vi "Return_EnFlo_Tunnel_to_Neutral.vi"(3 "Mode":T5, 5 "Traverse line In":T2 {"Carrier_2 Q (l/min)" format="%#.2f"; "Row Duration (mins)" format="%#.1f"; "Row No" min=0; "Trace Gas Concentration (%)" min=0.0 format="%#_4f"; "Carrier_1 Q (l/min)" format="%#.2f"; "Tunnel Speed" format="%#.2f"; "Start X" format="%#.2f"; "Start Y" format="%#.2f"; "Start Z" format="%#.2f"; "End X" format="%#.2f"; "End Y" format="%#.2f"; "End Z" format="%#.2f"; "Averaging time (min)" min=0.0 format="%#.2f"}) -> (0 "Error Message":string, 1 "Status":T1, 2 "Traverse line Out":T2 {"Carrier_2 Q (l/min)" format="%#.2f"; "Row Duration (mins)" format="%#.1f"; "Row No" min=0; "Trace Gas Concentration (%)" min=0.0 format="%#_4f"; "Carrier_1 Q (l/min)" format="%#.2f"; "Tunnel Speed" format="%#.2f"; "Start X" format="%#.2f"; "Start Y" format="%#.2f"; "Start Z" format="%#.2f"; "End X" format="%#.2f"; "End Y" format="%#.2f"; "End Z" format="%#.2f"; "Averaging time (min)" min=0.0 format="%#.2f"})   [LabVIEW 2016]
uses:
  Gen Trav/Traverse_cluster.ctl
  Gen Trav/Spacing.ctl
  Controls/Multi_run_mode.ctl
  Controls/User_Specific_mode.ctl
  Gen Trav/Multi_Run_Status.ctl
  ADAM Client/Sub VIs/ADAM Controls/Update_scan_value.ctl
  ADAM Client/Sub VIs/ADAM Controls/Channel_names.ctl
  ADAM Client/Sub VIs/ADAM Controls/Client_Source_Status.ctl
  Globals/Trav_pos_global.vi
panel:
  out "Chilled water supply temp":dbl(graph)
  # "X           Y            Z"
  # "Start"
  # "End"
  # "X           Y            Z"
  # "Start"
  # "End"
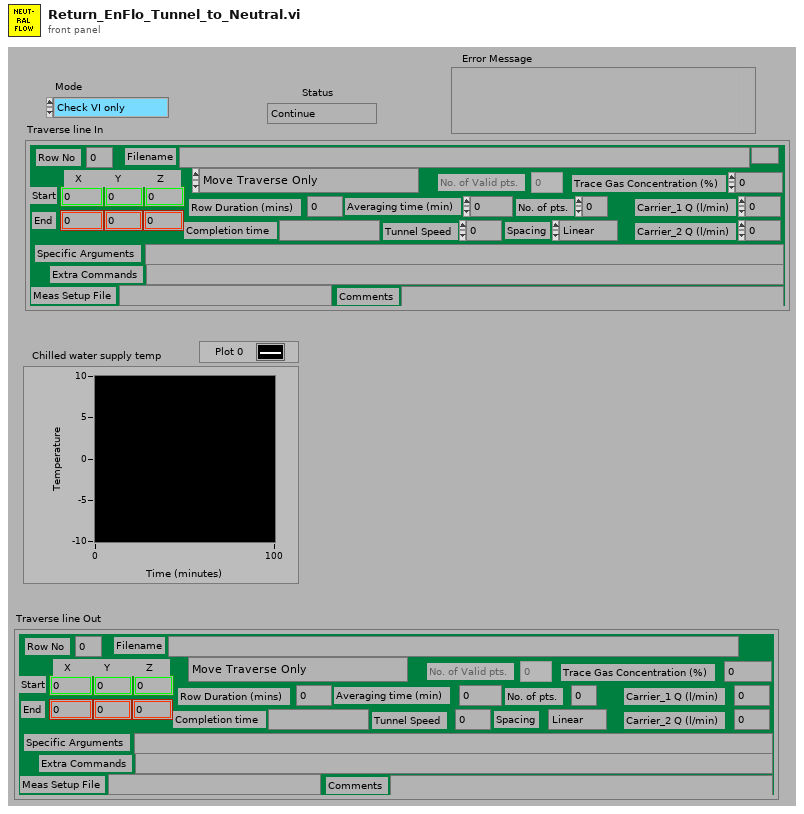
[diagram p1: front panel]
types:
  T1 = typedef "Multi_Run_Status.ctl" = enum16{"Continue", "Jump to Next Point", "Jump to Next Row", "Jump To Fall Back", "Terminate Run"}
  T2 = typedef "Traverse_cluster.ctl" = cluster{"Start X":sgl, "Start Y":sgl, "Start Z":sgl, "End X":sgl, "End Y":sgl, "End Z":sgl, "No. of pts.":i32, "Spacing":T3, "Filename":path, "Tunnel Speed":dbl, "Averaging time (min)":dbl, "Extra Commands":string, "Carrier_1 Q (l/min)":dbl, "Carrier_2 Q (l/min)":dbl, "Trace Gas Concentration (%)":dbl, "Specific Arguments":string, "Comments":string, "Row No":i32, "Row Type Selector":T4, "Completion time":string, "Row Duration (mins)":dbl, "No. of Valid pts.":i32, "Meas Setup File":string}
  T3 = typedef "Spacing.ctl" = enum16{"Linear", "Log", "Gauss", "Specified", "N/A"}
  T4 = typedef "Multi_run_mode.ctl" = enum16{"Move Traverse Only", "Set Tunnel Speed Only", "Set Source Only", "Set Measurement Conditions", "Single Measurement", "Vertical Profile", "Lateral Profile", "Longitudinal Profile", "Explore Volume", "Multi-Axis Profile", "Auto Calibrate", "Meas Fast FID Bkgnd", "Check Beam Power", "Scanning Valve Measurement", "Run VI Named:", "Set ADAM Ch", "Wait (minutes)", "Send Message", "Synchronize With:", "Fall Back to this Row", "Turn Off Row Repeating", "Blank Row", "Traverse 3D Volume"}
  T5 = typedef "User_Specific_mode.ctl" = enum16{"Check VI only", "Run VI"}
  T6 = typedef "Update_scan_value.ctl" = cluster{"Channel Name":string, "New Value":dbl}
  T7 = typedef "Channel_names.ctl" = enum16{"Active Only", "Active + Off", "All Channels"}
  T8 = typedef "Client_Source_Status.ctl" = enum16{"Not Using", "Using", "Must Have"}
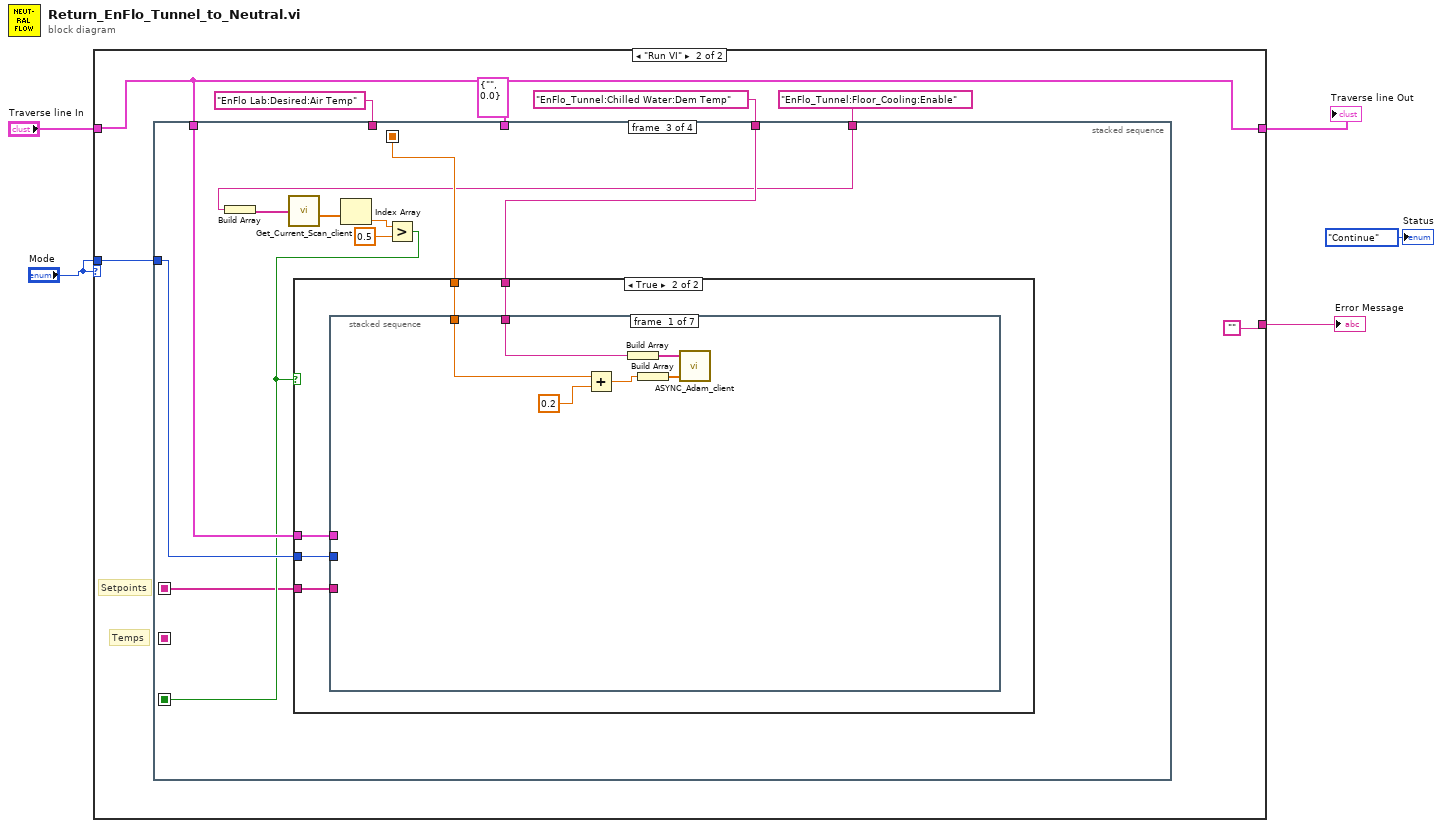
[diagram p0: block diagram]
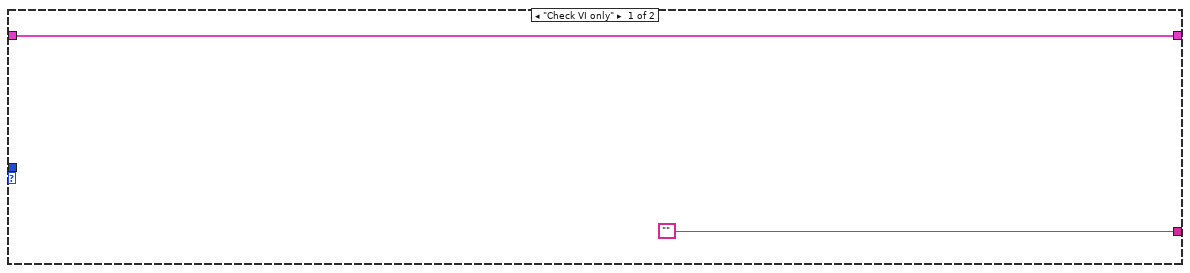
[diagram p2: hidden frame]
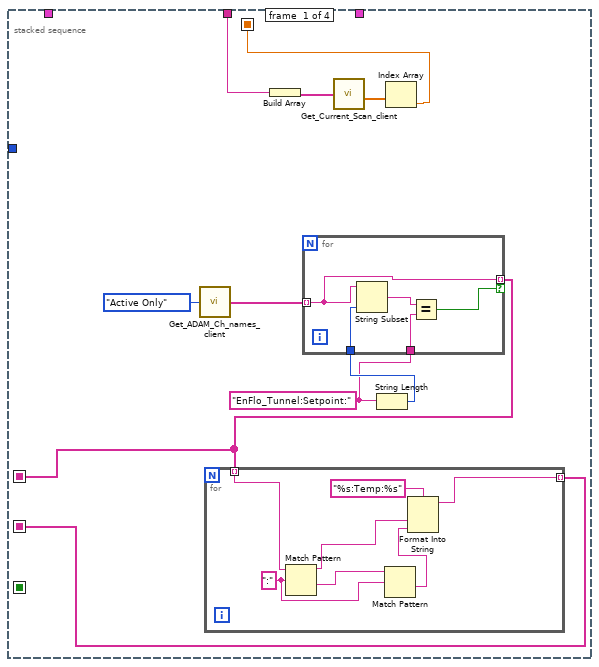
[diagram p3: hidden frame]
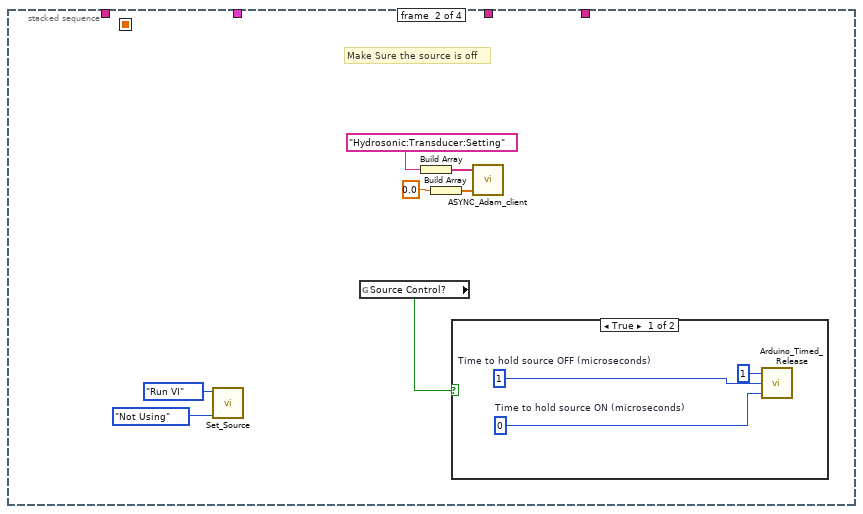
[diagram p4: hidden frame]
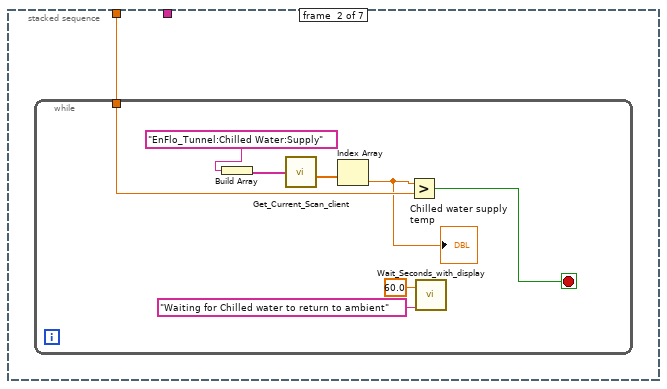
[diagram p7: hidden frame]
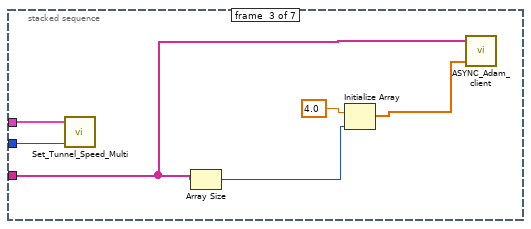
[diagram p8: hidden frame]
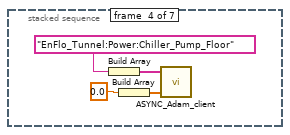
[diagram p9: hidden frame]
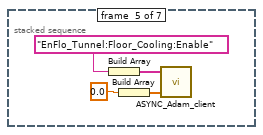
[diagram p10: hidden frame]
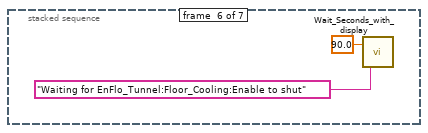
[diagram p11: hidden frame]
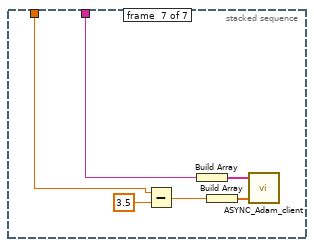
[diagram p12: hidden frame]
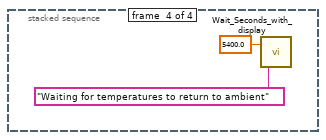
[diagram p13: hidden frame]
diagram:
  n1 = case shown="\"Run VI\"" "Mode" {
    tunnel: "Traverse line In" -> [w7 w12]
    tunnel: [w7 w12] -> w4
    tunnel: ["" ""] -> w3
    tunnel: "Mode" -> [_ w11]
    frame "Check VI only" {
    }
    frame "Run VI" {
      # "Setpoints"
      # "Temps"
      n2 = stacked-sequence {
        seq-local: [w17 _ _ _] -> [_ _ _ _]
        seq-local: [w15 _ _ _] -> [_ _ w56 _]
        seq-local: [_ _ w48 _] -> [_ _ _ _]
        seq-local: [w16 _ _ _] -> [_ _ w47 _]
        tunnel: T6 {"Channel Name"="", "New Value"=0.0} ("Update Scan Value Cluster") -> [_ _ _ _]
        tunnel: w12 -> [_ _ w55 _]
        tunnel: w11 -> [_ _ w54 _]
        tunnel: "EnFlo Lab:Desired:Air Temp" -> [w18 _ _ _]
        tunnel: "EnFlo_Tunnel:Chilled Water:Dem Temp" -> [_ _ w57 _]
        tunnel: "EnFlo_Tunnel:Floor_Cooling:Enable" -> [_ _ w49 _]
        frame #0 {
          w20 = "EnFlo_Tunnel:Setpoint:"
          n3 = call "Get_ADAM_Ch_names_client.vi"("Channel names set"=Channel_names."Active Only") -> ("Ch names"=w19:string[])
          n4 = Build Array(w18) -> (w24:string[])
          n5 = call "Get_Current_Scan_client.vi"("ADAM Ch Names"=w24) -> ("Numerical Values"=w23:dbl[])  [unwired: 1 in, 2 out]
          n6 = String Length(string=w20) -> (length=w21:i32)
          n7 = for {
            tunnel: w19 -> [w33] mode=indexing
            tunnel: w21 -> [w36]
            tunnel: w20 -> [w35]
            tunnel: [w33] -> w16 mode=indexing if=w32
            n8 = String Subset(string=w33, length (rest)=w36) -> (substring=w34:string)  [unwired: 1 out]
            n9 = Equal?(x=w34, y=w35) -> (x = y?=w32:bool)
          }
          n10 = for {
            tunnel: w16 -> [w25] mode=indexing
            tunnel: [w26] -> w17 mode=indexing
            w30 = ":" ("regular expression")
            n11 = Match Pattern(string=w25, regular expression=w30) -> (before substring=w28:string, after substring=w31:string)  [unwired: 3 out]
            n12 = Match Pattern(string=w31, regular expression=w30) -> (after substring=w27:string)  [unwired: 4 out]
            n13 = Format Into String(format string="%s:Temp:%s", w28, w27) -> (resulting string=w26:string)  [unwired: 2 in, 1 out]
          }
          n14 = Index Array(array=w23) -> (element=w15:dbl)  [unwired: 1 in]
        }
        frame #1 {
          # "Make Sure the source is off"
          n15 = call "Set_Source.vi"("Source Status"=Client_Source_Status."Not Using", "Simulate/Run"=User_Specific_mode."Run VI") -> ()  [unwired: 2 in, 6 out]
          n16 = global read "Trav_pos_global.vi" "Source Control?"() -> (w41:bool)
          n17 = Build Array("Hydrosonic:Transducer:Setting") -> (w38:string[])
          n18 = Build Array(0.0 ("element")) -> (w39:dbl[])
          n19 = case shown="True" w41 {
            frame True {
              w45 = u32 1  # Time to hold source OFF (microseconds)
              w44 = u32 0  # Time to hold source ON (microseconds)
              n20 = call "Arduino_Timed_Release.vi"("Time to hold source ON (microseconds)"=w44, "Time to hold source OFF (microseconds)"=w45, "Number of cycles"=u16 1) -> ()  [unwired: 2 out]
            }
            frame False {
            }
          }
          n21 = call "ASYNC_Adam_client.vi"("Values"=w39, "Channel Names"=w38) -> ()  [unwired: 1 in, 2 out]
        }
        frame #2 {
          n22 = Build Array(w49) -> (w52:string[])
          n23 = call "Get_Current_Scan_client.vi"("ADAM Ch Names"=w52) -> ("Numerical Values"=w53:dbl[])  [unwired: 1 in, 2 out]
          n24 = Index Array(array=w53) -> (element=w51:dbl)  [unwired: 1 in]
          n25 = Greater?(x=w51, y=0.5) -> (0:w48:bool)
          n26 = case shown="True" w48 {
            tunnel: w57 -> [_ w59]
            tunnel: w56 -> [_ w60]
            tunnel: w55 -> [_ w62]
            tunnel: w54 -> [_ w61]
            tunnel: w47 -> [_ w58]
            frame False {
            }
            frame True {
              n27 = stacked-sequence {
                tunnel: w62 -> [_ _ w79 _ _ _ _]
                tunnel: w61 -> [_ _ w78 _ _ _ _]
                tunnel: w60 -> [w65 w69 _ _ _ _ w94]
                tunnel: w59 -> [w66 _ _ _ _ _ w95]
                tunnel: w58 -> [_ _ w80 _ _ _ _]
                frame #0 {
                  n28 = Add(x=w65, y=0.2) -> (x+y=w64:dbl)
                  n29 = Build Array(w66) -> (w67:string[])
                  n30 = Build Array(w64) -> (w68:dbl[])
                  n31 = call "ASYNC_Adam_client.vi"("Values"=w68, "Channel Names"=w67) -> ()  [unwired: 1 in, 2 out]
                }
                frame #1 {
                  n32 = while {
                    tunnel: w69 -> [w75]
                    stop <- w74 stop-if-true
                    n33 = Build Array("EnFlo_Tunnel:Chilled Water:Supply") -> (w77:string[])
                    n34 = call "Get_Current_Scan_client.vi"("ADAM Ch Names"=w77) -> ("Numerical Values"=w76:dbl[])  [unwired: 1 in, 2 out]
                    n35 = Index Array(array=w76) -> (element=w70:dbl)  [unwired: 1 in]
                    "Chilled water supply temp" <- w70
                    n36 = Greater?(x=w70, y=w75) -> (0:w74:bool)
                    n37 = call "Wait_Seconds_with_display.vi"("Message"="Waiting for Chilled water to return to ambient", "Seconds to wait"=60.0) -> ()  [unwired: 1 in, 1 out]
                  }
                }
                frame #2 {
                  n38 = call "Set_Tunnel_Speed_Multi.vi"("Simulate/Run"=w78, "Traverse line"=w79) -> ()  [unwired: 4 out]
                  n39 = Array Size(array=w80) -> (size(s)=w83:i32)
                  n40 = Initialize Array(4.0 ("Input Element"), w83) -> (w81:dbl[])
                  n41 = call "ASYNC_Adam_client.vi"("Values"=w81, "Channel Names"=w80) -> ()  [unwired: 1 in, 2 out]
                }
                frame #3 {
                  n42 = Build Array("EnFlo_Tunnel:Power:Chiller_Pump_Floor") -> (w86:string[])
                  n43 = Build Array(0.0 ("element")) -> (w85:dbl[])
                  n44 = call "ASYNC_Adam_client.vi"("Values"=w85, "Channel Names"=w86) -> ()  [unwired: 1 in, 2 out]
                }
                frame #4 {
                  n45 = Build Array("EnFlo_Tunnel:Floor_Cooling:Enable") -> (w89:string[])
                  n46 = Build Array(0.0 ("element")) -> (w90:dbl[])
                  n47 = call "ASYNC_Adam_client.vi"("Values"=w90, "Channel Names"=w89) -> ()  [unwired: 1 in, 2 out]
                }
                frame #5 {
                  n48 = call "Wait_Seconds_with_display.vi"("Message"="Waiting for EnFlo_Tunnel:Floor_Cooling:Enable to shut", "Seconds to wait"=90.0) -> ()  [unwired: 1 in, 1 out]
                }
                frame #6 {
                  n49 = Subtract(x=w94, y=3.5) -> (x-y=w96:dbl)
                  n50 = Build Array(w95) -> (w99:string[])
                  n51 = Build Array(w96) -> (w98:dbl[])
                  n52 = call "ASYNC_Adam_client.vi"("Values"=w98, "Channel Names"=w99) -> ()  [unwired: 1 in, 2 out]
                }
              }
            }
          }
        }
        frame #3 {
          n53 = call "Wait_Seconds_with_display.vi"("Message"="Waiting for temperatures to return to ambient", "Seconds to wait"=5400.0) -> ()  [unwired: 1 in, 1 out]
        }
      }
    }
  }
  "Traverse line Out" <- w4
  "Error Message" <- w3
  "Status" <- Multi_Run_Status."Continue" ("Status")
